vi "angle obtained for rotation.vi"(9 "Search Direction":enum16{"Horizontal", "Vertical"}(ring)=enum."Vertical", 10 "Angle (deg) System":sgl, 11 "Angle (deg) Obtained":sgl) -> (3 "Total Rotation":dbl)   [LabVIEW 2014]
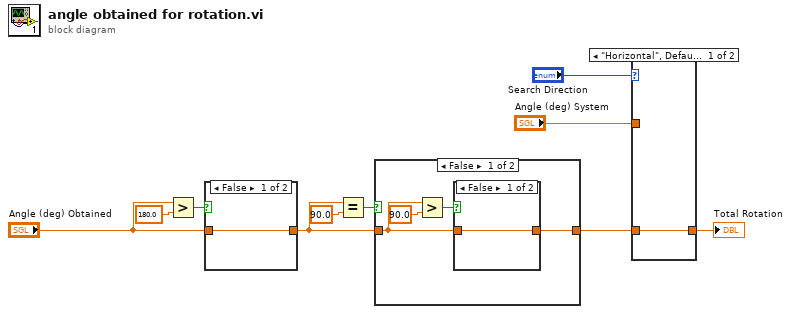
[diagram p0: block diagram]
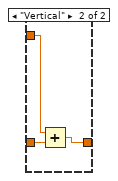
[diagram p2: hidden frame]
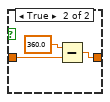
[diagram p3: hidden frame]
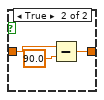
[diagram p4: hidden frame]
diagram:
  n1 = Greater?(x="Angle (deg) Obtained", y=sgl 180.0) -> (0:w2:bool)
  n2 = case shown="False" w2 {
    tunnel: [w11 w14] -> w7
    tunnel: "Angle (deg) Obtained" -> [w11 w12]
    frame False {
    }
    frame True {
      n3 = Subtract(x=sgl 360.0, y=w12) -> (x-y=w14:sgl)
    }
  }
  n4 = Equal?(x=w7, y=sgl 90.0) -> (x = y?=w6:bool)
  n5 = case shown="False" w6 {
    tunnel: w7 -> [w16 w23]
    tunnel: [w15 w23] -> w9
    frame False {
      n6 = Greater?(x=w16, y=sgl 90.0) -> (0:w17:bool)
      n7 = case shown="False" w17 {
        tunnel: w16 -> [w19 w22]
        tunnel: [w19 w20] -> w15
        frame False {
        }
        frame True {
          n8 = Subtract(x=w22, y=sgl 90.0) -> (x-y=w20:sgl)
        }
      }
    }
    frame True {
    }
  }
  n9 = case shown="\"Horizontal\", Default" "Search Direction" {
    tunnel: [w24 w27] -> w10
    tunnel: w9 -> [w24 w26]
    tunnel: "Angle (deg) System" -> [_ w25]
    frame "Horizontal", Default {
    }
    frame "Vertical" {
      n10 = Add(x=w25, y=w26) -> (x+y=w27:sgl)
    }
  }
  "Total Rotation" <- w10
